vi "PositionControlsGen.vi"(6 "Horizontal(T)":bool=TRUE, 8 "ErrorIn(No Error)":errorcluster caption="entrée d'erreur (pas d'erreur)", 9 "Position":T1, 10 "Limites":T2, 11 "FA_Ref":refnum<vi>[](array[refnum])) -> (0 "sortie d'erreur":errorcluster)   [LabVIEW 2010]
uses:
  <vilib>/Utility/miscctls.llb/LVBoundsTypeDef.ctl
  <vilib>/Utility/miscctls.llb/LVPositionTypeDef.ctl
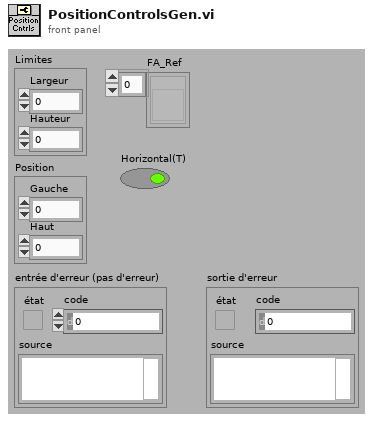
[diagram p1: front panel]
types:
  T1 = typedef "LVPositionTypeDef.ctl" = cluster{"Left":i32, "Top":i32}
  T2 = typedef "LVBoundsTypeDef.ctl" = cluster{"Width":u32, "Height":u32}
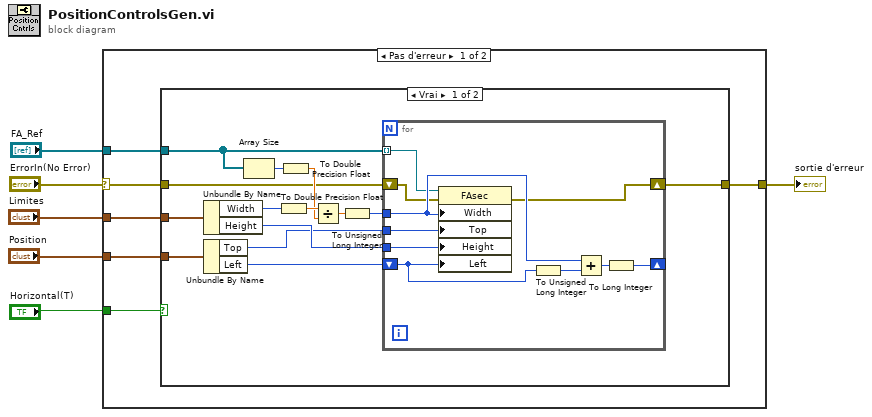
[diagram p0: block diagram]
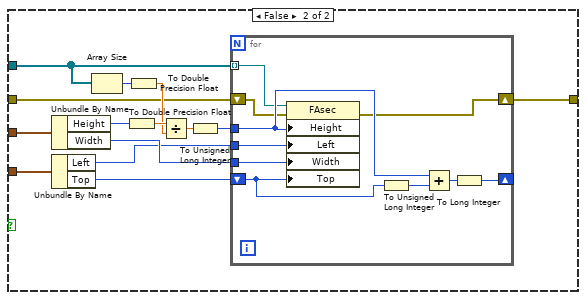
[diagram p2: hidden frame]
diagram:
  n1 = case shown="Pas d'erreur" "ErrorIn(No Error)" {
    selector: "ErrorIn(No Error)" -> [w8 w61]
    tunnel: [w7 w61] -> w5
    tunnel: "FA_Ref" -> [w12 _]
    tunnel: "Limites" -> [w11 _]
    tunnel: "Position" -> [w10 _]
    tunnel: "Horizontal(T)" -> [w9 _]
    frame No Error {
      n2 = case shown="Vrai" w9 {
        tunnel: w12 -> [w21 w45]
        tunnel: w11 -> [w20 w44]
        tunnel: w10 -> [w17 w41]
        tunnel: w8 -> [w14 w38]
        tunnel: [w13 w37] -> w7
        frame True {
          n3 = Unbundle By Name(w20) -> ("Width"=w19:u32, "Height"=w18:u32)
          n4 = Unbundle By Name(w17) -> ("Top"=w15:i32, "Left"=w16:i32)
          n5 = Array Size(array=w21) -> (size(s)=w24:i32)
          n6 = To Double Precision Float(number=w19) -> (double precision float=w25:dbl)
          n7 = To Double Precision Float(number=w24) -> (double precision float=w23:dbl)
          n8 = Divide(x=w25, y=w23) -> (x/y=w26:dbl)
          n9 = To Unsigned Long Integer(number=w26) -> (unsigned 32bit integer=w22:u32)
          n10 = for {
            tunnel: w21 -> [w29] mode=indexing
            tunnel: w18 -> [w35]
            tunnel: w15 -> [w34]
            shift-right: [w33] -> _
            shift-left: w16 -> [w31]
            tunnel: w22 -> [w30]
            shift-right: [w27] -> w13
            shift-left: w14 -> [w28]
            n11 = property class="FAsec"(reference=w29, error in=w28, "Width"=w30, "Top"=w34, "Height"=w35, "Left"=w31) -> (error out=w27:errorcluster)  [unwired: 1 out]
            n12 = To Unsigned Long Integer(number=w31) -> (unsigned 32bit integer=w32:u32)
            n13 = Add(x=w30, y=w32) -> (x+y=w36:u32)
            n14 = To Long Integer(number=w36) -> (32bit integer=w33:i32)
          }
        }
        frame False {
          n15 = Unbundle By Name(w44) -> ("Height"=w43:u32, "Width"=w42:u32)
          n16 = Unbundle By Name(w41) -> ("Left"=w39:i32, "Top"=w40:i32)
          n17 = Array Size(array=w45) -> (size(s)=w48:i32)
          n18 = To Double Precision Float(number=w43) -> (double precision float=w49:dbl)
          n19 = To Double Precision Float(number=w48) -> (double precision float=w47:dbl)
          n20 = Divide(x=w49, y=w47) -> (x/y=w50:dbl)
          n21 = To Unsigned Long Integer(number=w50) -> (unsigned 32bit integer=w46:u32)
          n22 = for {
            tunnel: w45 -> [w53] mode=indexing
            tunnel: w42 -> [w59]
            tunnel: w39 -> [w58]
            shift-right: [w57] -> _
            shift-left: w40 -> [w55]
            tunnel: w46 -> [w54]
            shift-right: [w51] -> w37
            shift-left: w38 -> [w52]
            n23 = property class="FAsec"(reference=w53, error in=w52, "Height"=w54, "Left"=w58, "Width"=w59, "Top"=w55) -> (error out=w51:errorcluster)  [unwired: 1 out]
            n24 = To Unsigned Long Integer(number=w55) -> (unsigned 32bit integer=w56:u32)
            n25 = Add(x=w54, y=w56) -> (x+y=w60:u32)
            n26 = To Long Integer(number=w60) -> (32bit integer=w57:i32)
          }
        }
      }
    }
    frame Error {
    }
  }
  "sortie d'erreur" <- w5
